vi "dispose server acceptor.vi"(8 "error in":errorcluster, 11 "acceptor":u64) -> (0 "error out":errorcluster)   [LabVIEW 2016]
uses:
  async tls dl.lvlib
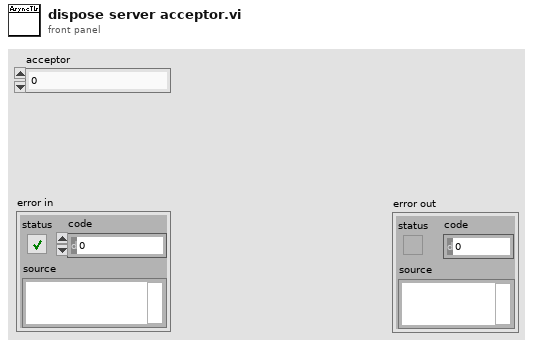
[diagram p1: front panel]
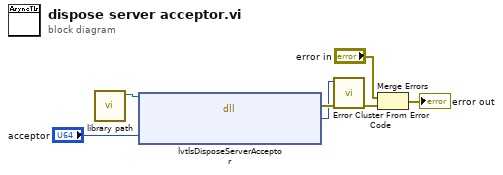
[diagram p0: block diagram]
diagram:
  n1 = call "library path.vi"() -> ("path"=w1:path)  [unwired: 11 in]
  n2 = dll-call lib="C:/Users/IEUser/Desktop/libasynclvtls/lvasynctls.dll" fn="lvtlsDisposeServerAcceptor"(path in=w1, "acceptor"="acceptor") -> (error out=w7:errorcluster, "err"=w6:i32)  [unwired: 3 in, 1 out]
  n3 = call <vilib>:"Error Cluster From Error Code.vi"("error in (no error)"=w7, "error code (0)"=w6) -> ("error out"=w4:errorcluster)  [unwired: 7 in]
  n4 = Merge Errors("error in", w4) -> (→"error out":errorcluster)
